vi "CRC_MOD.vi"(1 "输入":bool[](array[boolean])) -> (0 "输出":bool[](array[boolean]))   [LabVIEW 2015]
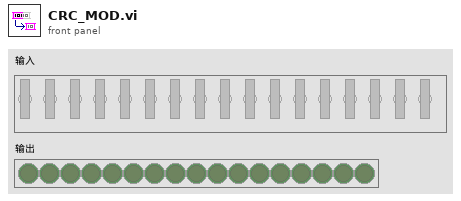
[diagram p1: front panel]
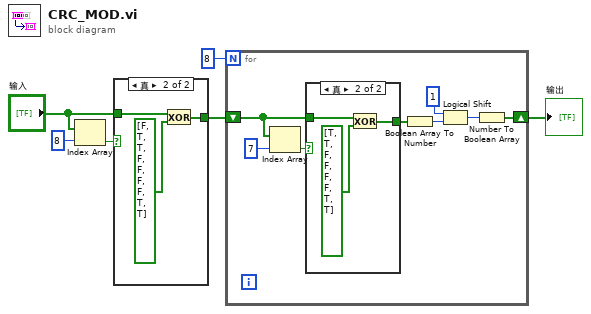
[diagram p0: block diagram]
diagram:
  n1 = Index Array(array="输入", index=8) -> (element=w4:bool)
  n2 = case shown="真" w4 {
    tunnel: "输入" -> [w7 w10]
    tunnel: [w7 w9] -> w3
    frame False {
    }
    frame True {
      n3 = Exclusive Or(1:bool[] [FALSE, TRUE, TRUE, FALSE, FALSE, FALSE, FALSE, TRUE, TRUE], 2:w10) -> (0:w9:bool[])
    }
  }
  n4 = for {
    N: 8 -> [_]
    shift-right: [w11] -> w1
    shift-left: w3 -> [w15]
    n5 = Index Array(array=w15, index=7) -> (element=w17:bool)
    n6 = case shown="真" w17 {
      tunnel: [w19 w21] -> w14
      tunnel: w15 -> [w19 w22]
      frame False {
      }
      frame True {
        n7 = Exclusive Or(1:bool[] [TRUE, TRUE, FALSE, FALSE, FALSE, FALSE, TRUE, TRUE], 2:w22) -> (0:w21:bool[])
      }
    }
    n8 = Boolean Array To Number(Boolean array=w14) -> (number=w13:u32)
    n9 = Logical Shift(y=1, x=w13) -> (x << y=w12:u32)
    n10 = Number To Boolean Array(number=w12) -> (Boolean array=w11:bool[])
  }
  "输出" <- w1
